vi "Main.vi"() -> ()   [LabVIEW 2017]
uses:
  states.ctl
  data.ctl
panel:
  in  "Save Config":bool caption="Save"
  in  "Log While\nCharging":enum32{"No Selection", " Yes", " No"}(radio) caption="Radio Buttons"
  in  "Sample\nRate":T1(radio) caption="Radio Buttons"
  in  "Load Config":bool caption="Config"
  in  "Download All (Single)":bool
  in  "Download File Path":path
  in  "Download":bool
  in  "View File":bool
  in  "File Selection":u16(ring)
  in  "Drifter Selection":u16(ring) items=["Drifter Number: 000 (10.0.1.3)", "Drifter Number: 001 (10.0.1.6)"]
  out "Info Box":string
  in  "Save Table":bool
  in  "Load Table":bool
  in  "MAC & Name":string[][](table)=[["", ""], ["", ""]]
  in  "Find Drifters":bool
  in  "List Data Files":bool
  in  "Stop":bool
  # "GPS Drifter Interface Software"
  # "Wolfson School of Mechanical, Electrical and Manufacturing Engineering"
  # "Thomas Quinn B224307 MEng Advanced Project 2017/2018"
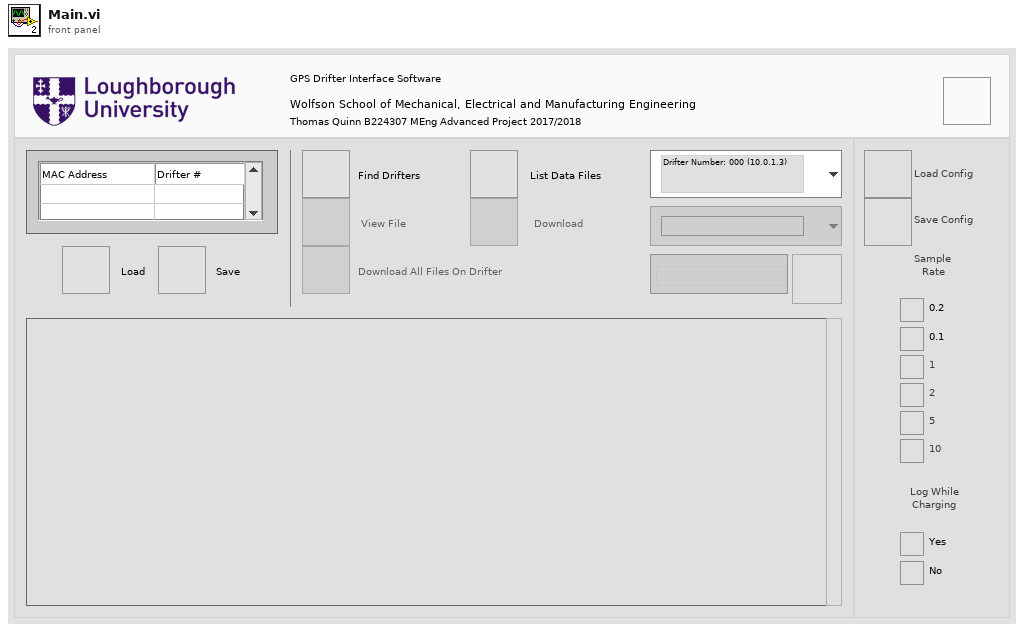
[diagram p1: front panel]
types:
  T1 = enum32{"No Selection", " 0.2", " 0.1", " 1", " 2", " 5", " 10"}
  T2 = enum8{"Enabled", "Disabled", "Disabled and Grayed Out"}
  T3 = typedef "data.ctl" = cluster{"Info Box":string, "MAC & Name Out":string[][], "Default Gateway":string, "Drfiter IP Addresses":string[][], "Network Map":string, "Drifter Selection":i32, "File Selection":i32, "Download File Path":path, "File Selection Strings":string[], "Sample Rate":enum32{"No Selection", " 0.2", " 0.1", " 1", " 2", " 5", " 10"}, "Log While Charging":enum32{"No Selection", " Yes", " No"}}
  T4 = typedef "states.ctl" = cluster{"Enum":enum16{"Stop", "Init", "List Data Files", "Find Default Gateway", "Save Table", "Load Table", "Ping Entire Network", "Network Map", "Match MAC Addresses", "Check IP Addresses", "Display IP Addresses", "File Selection", "View File", "Download File", "Download All (Single)", "Download File Path", "Load Config", "Save Config", "Update Config"}, "Message Data":variant}
  T5 = enum16{"Stop", "Init", "List Data Files", "Find Default Gateway", "Save Table", "Load Table", "Ping Entire Network", "Network Map", "Match MAC Addresses", "Check IP Addresses", "Display IP Addresses", "File Selection", "View File", "Download File", "Download All (Single)", "Download File Path", "Load Config", "Save Config", "Update Config"}
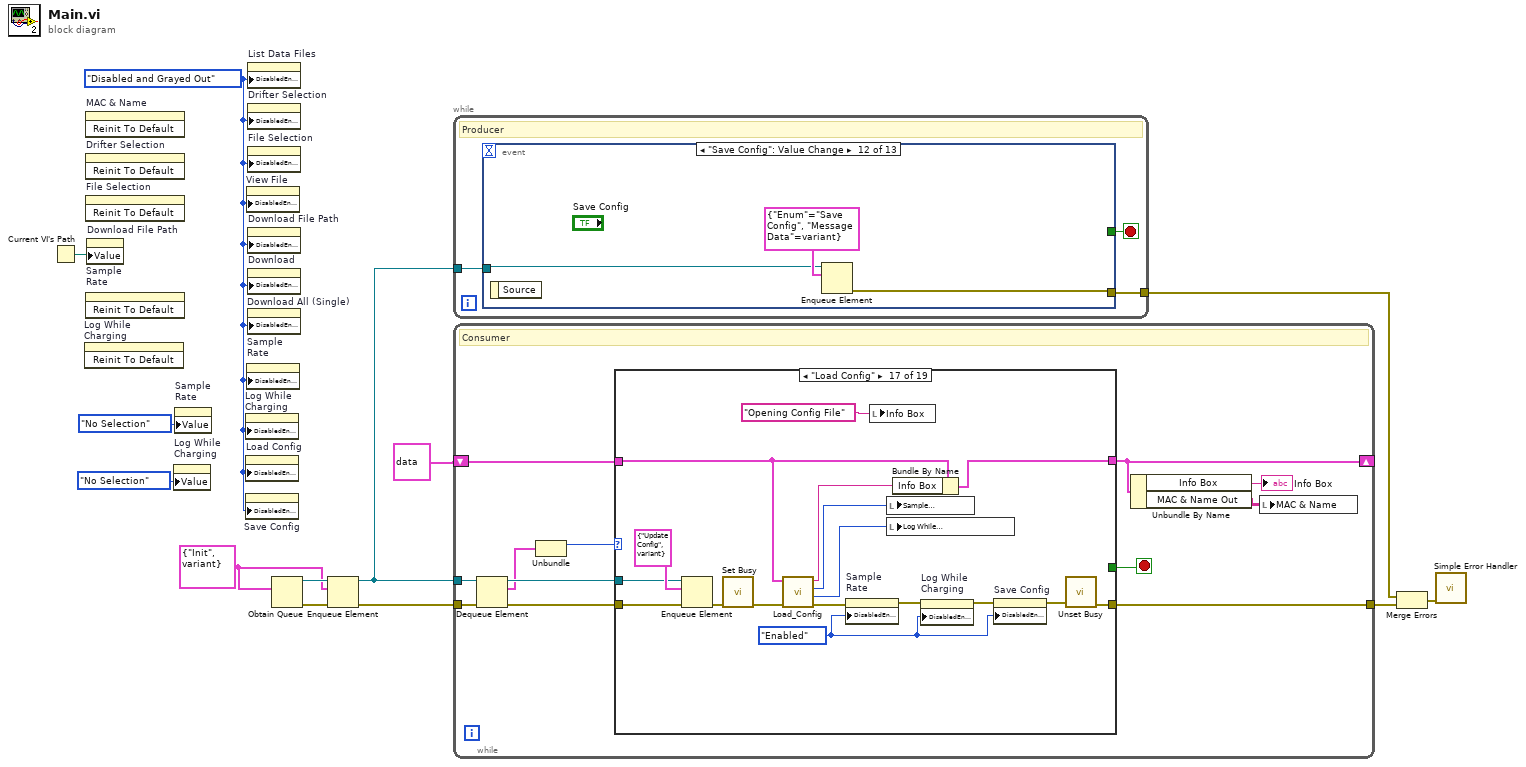
[diagram p0: block diagram]
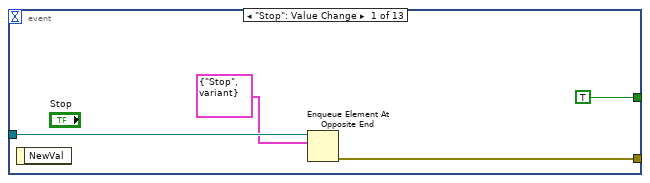
[diagram p2: hidden frame]
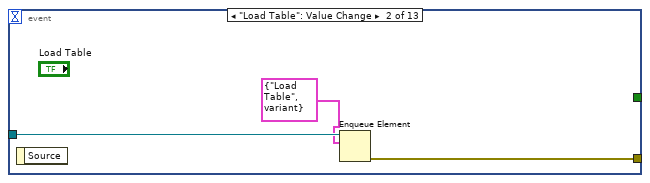
[diagram p3: hidden frame]
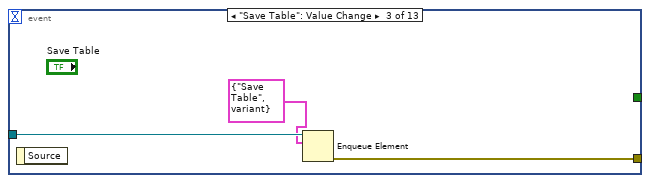
[diagram p4: hidden frame]
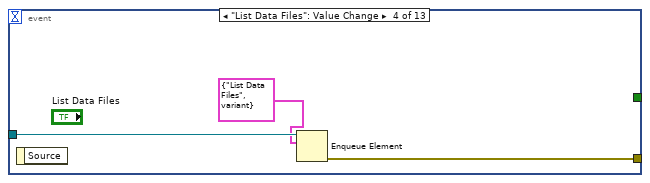
[diagram p5: hidden frame]
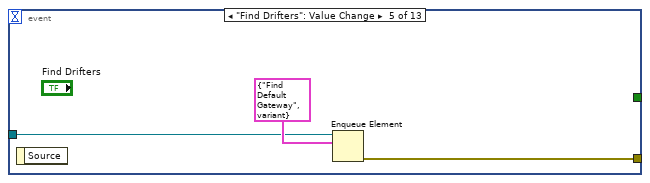
[diagram p6: hidden frame]
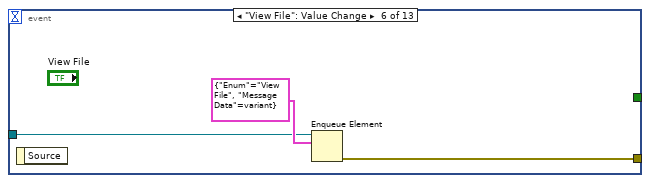
[diagram p7: hidden frame]
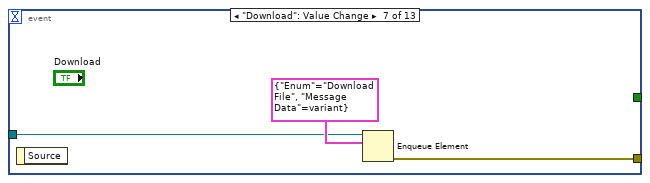
[diagram p8: hidden frame]
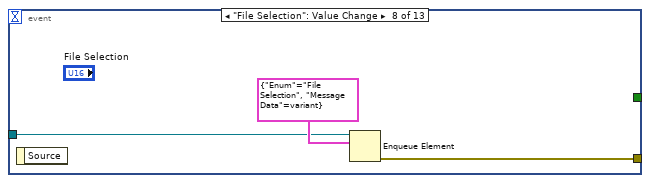
[diagram p9: hidden frame]
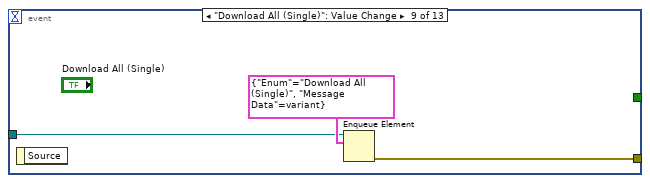
[diagram p10: hidden frame]
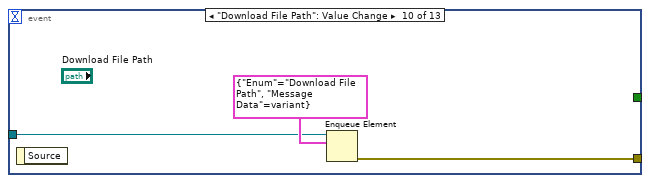
[diagram p11: hidden frame]
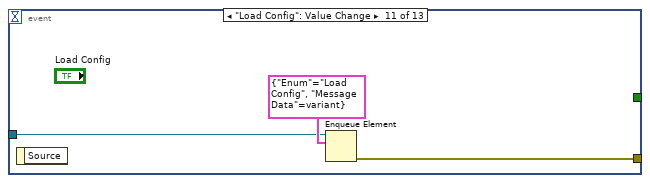
[diagram p12: hidden frame]
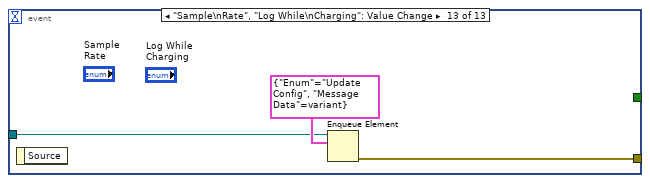
[diagram p13: hidden frame]
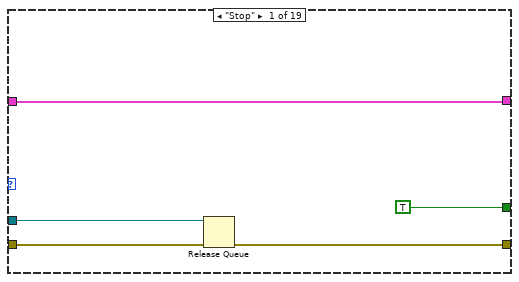
[diagram p14: hidden frame]
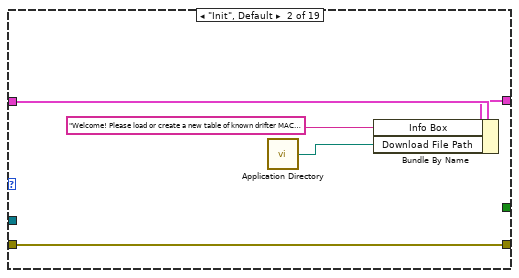
[diagram p15: hidden frame]
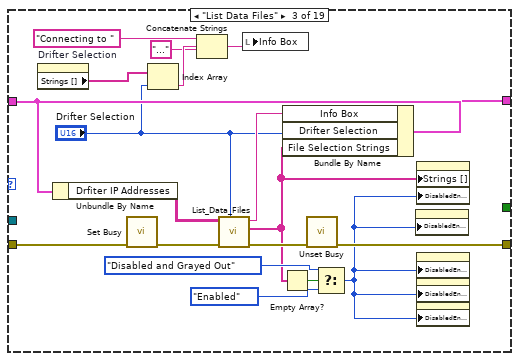
[diagram p16: hidden frame]
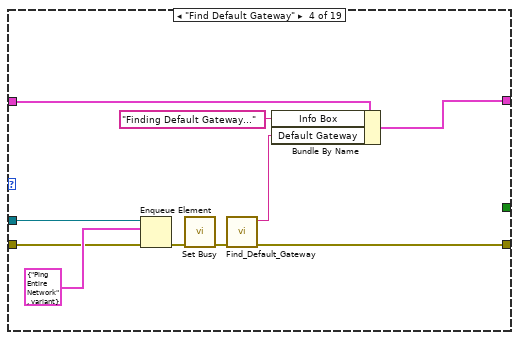
[diagram p17: hidden frame]
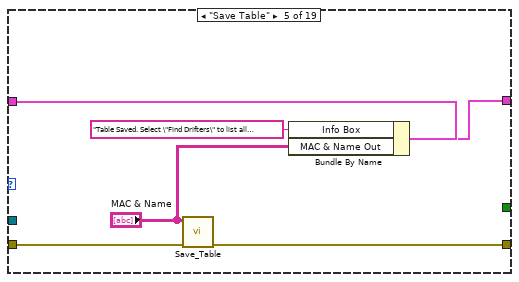
[diagram p18: hidden frame]
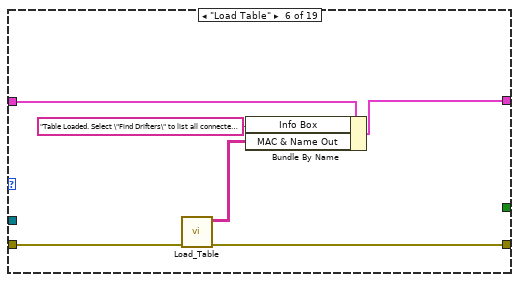
[diagram p19: hidden frame]
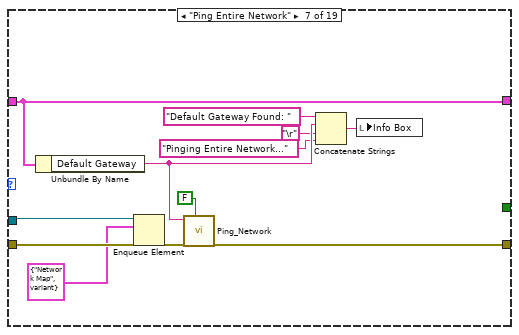
[diagram p20: hidden frame]
diagram:
  w1 = T2."Disabled and Grayed Out" ("Disabled")
  w6 = T4 {"Enum"=enum."Init", "Message Data"=variant}
  n1 = Current VI's Path() -> (path=w4:path)
  n2 = invoke on="Log While\nCharging" class="RadioBtnsControl (strict)" method="Reinit To Default"() -> ()  [unwired: 3 in, 3 out]
  n3 = invoke on="MAC & Name" class="Tbl (strict)" method="Reinit To Default"() -> ()  [unwired: 3 in, 3 out]
  n4 = invoke on="Drifter Selection" class="Ring (strict)" method="Reinit To Default"() -> ()  [unwired: 3 in, 3 out]
  n5 = invoke on="File Selection" class="Ring (strict)" method="Reinit To Default"() -> ()  [unwired: 3 in, 3 out]
  n6 = invoke on="Sample\nRate" class="RadioBtnsControl (strict)" method="Reinit To Default"() -> ()  [unwired: 3 in, 3 out]
  n7 = property on="Download File Path" class="Path"("Value"=w4) -> ()  [unwired: 2 in, 2 out]
  n8 = property on="Log While\nCharging" class="RadioBtnsControl (strict)"("Value"=enum32{"No Selection", " Yes", " No"}."No Selection" ("Log While\nCharging")) -> ()  [unwired: 2 in, 2 out]
  n9 = property on="Sample\nRate" class="RadioBtnsControl (strict)"("Value"=T1."No Selection" ("Sample\nRate")) -> ()  [unwired: 2 in, 2 out]
  n10 = property on="Log While\nCharging" class="RadioBtnsControl (strict)"("DisabledEnum"=w1) -> ()  [unwired: 2 in, 2 out]
  n11 = property on="Load Config" class="Bool"("DisabledEnum"=w1) -> ()  [unwired: 2 in, 2 out]
  n12 = property on="Save Config" class="Bool"("DisabledEnum"=w1) -> ()  [unwired: 2 in, 2 out]
  n13 = property on="View File" class="Bool"("DisabledEnum"=w1) -> ()  [unwired: 2 in, 2 out]
  n14 = property on="Sample\nRate" class="RadioBtnsControl (strict)"("DisabledEnum"=w1) -> ()  [unwired: 2 in, 2 out]
  n15 = property on="List Data Files" class="Bool"("DisabledEnum"=w1) -> ()  [unwired: 2 in, 2 out]
  n16 = property on="Drifter Selection" class="Ring (strict)"("DisabledEnum"=w1) -> ()  [unwired: 2 in, 2 out]
  n17 = property on="File Selection" class="Ring (strict)"("DisabledEnum"=w1) -> ()  [unwired: 2 in, 2 out]
  n18 = property on="Download File Path" class="Path"("DisabledEnum"=w1) -> ()  [unwired: 2 in, 2 out]
  n19 = property on="Download" class="Bool"("DisabledEnum"=w1) -> ()  [unwired: 2 in, 2 out]
  n20 = property on="Download All (Single)" class="Bool"("DisabledEnum"=w1) -> ()  [unwired: 2 in, 2 out]
  n21 = Obtain Queue(element data type=w6) -> (queue out=w10:refnum<queue>, error out=w11:errorcluster)  [unwired: 4 in, 1 out]
  n22 = Enqueue Element(queue=w10, element=w6, error in (no error)=w11) -> (queue out=w8:refnum<queue>, error out=w9:errorcluster)  [unwired: 1 in, 1 out]
  n23 = while {
    tunnel: w8 -> [w16]
    tunnel: [w14] -> w12
    stop <- w15 stop-if-true
    # "Producer"
    n24 = event shown="[11] \"Save Config\": Value Change" {
      selector: _ -> [_ _ _ _ _ _ _ _ _ _ _ _ _]
      dyn-events: _ -> [_ _ _ _ _ _ _ _ _ _ _ _ _]
      timeout: _ -> [_ _ _ _ _ _ _ _ _ _ _ _ _]
      tunnel: [TRUE _ _ _ _ _ _ _ _ _ _ _ _] -> w15
      tunnel: w16 -> [w20 w22 w25 w28 w31 w33 w36 w39 w42 w45 w48 w51 w54]
      tunnel: [w19 w23 w26 w29 w30 w34 w37 w40 w43 w46 w49 w52 w55] -> w14
      event "Stop": Value Change {
        n25 = event-data() -> ()  [unwired: 1 in, 1 out]
        n26 = Enqueue Element At Opposite End(queue=w20, element=T4 {"Enum"=enum."Stop", "Message Data"=variant}) -> (error out=w19:errorcluster)  [unwired: 2 in, 2 out]
      }
      event "Load Table": Value Change {
        n27 = event-data() -> ()  [unwired: 1 in, 1 out]
        n28 = Enqueue Element(queue=w22, element=T4 {"Enum"=enum."Load Table", "Message Data"=variant}) -> (error out=w23:errorcluster)  [unwired: 2 in, 2 out]
      }
      event "Save Table": Value Change {
        n29 = event-data() -> ()  [unwired: 1 in, 1 out]
        n30 = Enqueue Element(queue=w25, element=T4 {"Enum"=enum."Save Table", "Message Data"=variant}) -> (error out=w26:errorcluster)  [unwired: 2 in, 2 out]
      }
      event "List Data Files": Value Change {
        n31 = event-data() -> ()  [unwired: 1 in, 1 out]
        n32 = Enqueue Element(queue=w28, element=T4 {"Enum"=enum."List Data Files", "Message Data"=variant}) -> (error out=w29:errorcluster)  [unwired: 2 in, 2 out]
      }
      event "Find Drifters": Value Change {
        n33 = event-data() -> ()  [unwired: 1 in, 1 out]
        n34 = Enqueue Element(queue=w31, element=T4 {"Enum"=enum."Find Default Gateway", "Message Data"=variant}) -> (error out=w30:errorcluster)  [unwired: 2 in, 2 out]
      }
      event "View File": Value Change {
        n35 = event-data() -> ()  [unwired: 1 in, 1 out]
        n36 = Enqueue Element(queue=w33, element=T4 {"Enum"=enum."View File", "Message Data"=variant}) -> (error out=w34:errorcluster)  [unwired: 2 in, 2 out]
      }
      event "Download": Value Change {
        n37 = event-data() -> ()  [unwired: 1 in, 1 out]
        n38 = Enqueue Element(queue=w36, element=T4 {"Enum"=enum."Download File", "Message Data"=variant}) -> (error out=w37:errorcluster)  [unwired: 2 in, 2 out]
      }
      event "File Selection": Value Change {
        n39 = event-data() -> ()  [unwired: 1 in, 1 out]
        n40 = Enqueue Element(queue=w39, element=T4 {"Enum"=enum."File Selection", "Message Data"=variant}) -> (error out=w40:errorcluster)  [unwired: 2 in, 2 out]
      }
      event "Download All (Single)": Value Change {
        n41 = event-data() -> ()  [unwired: 1 in, 1 out]
        n42 = Enqueue Element(queue=w42, element=T4 {"Enum"=enum."Download All (Single)", "Message Data"=variant}) -> (error out=w43:errorcluster)  [unwired: 2 in, 2 out]
      }
      event "Download File Path": Value Change {
        n43 = event-data() -> ()  [unwired: 1 in, 1 out]
        n44 = Enqueue Element(queue=w45, element=T4 {"Enum"=enum."Download File Path", "Message Data"=variant}) -> (error out=w46:errorcluster)  [unwired: 2 in, 2 out]
      }
      event "Load Config": Value Change {
        n45 = event-data() -> ()  [unwired: 1 in, 1 out]
        n46 = Enqueue Element(queue=w48, element=T4 {"Enum"=enum."Load Config", "Message Data"=variant}) -> (error out=w49:errorcluster)  [unwired: 2 in, 2 out]
      }
      event "Save Config": Value Change {
        n47 = event-data() -> ()  [unwired: 1 in, 1 out]
        n48 = Enqueue Element(queue=w51, element=T4 {"Enum"=enum."Save Config", "Message Data"=variant}) -> (error out=w52:errorcluster)  [unwired: 2 in, 2 out]
      }
      event "Sample\nRate", "Log While\nCharging": Value Change {
        n49 = event-data() -> ()  [unwired: 1 in, 1 out]
        n50 = Enqueue Element(queue=w54, element=T4 {"Enum"=enum."Update Config", "Message Data"=variant}) -> (error out=w55:errorcluster)  [unwired: 2 in, 2 out]
      }
    }
  }
  n51 = while {
    tunnel: w8 -> [w66]
    tunnel: w9 -> [w67]
    tunnel: [w68] -> w13
    shift-right: [w59] -> _
    shift-left: T3 {"Info Box"="", "MAC & Name Out"=[], "Default Gateway"="", "Drfiter IP Addresses"=[], "Network Map"="", "Drifter Selection"=0, "File Selection"=0, "Download File Path"=path "", "File Selection Strings"=[], "Sample Rate"=enum." 0.2", "Log While Charging"=enum." Yes"} ("Data") -> [w60]
    stop <- w61 stop-if-true
    # "Consumer"
    n52 = Dequeue Element(queue=w66, error in (no error)=w67) -> (queue out=w65:refnum<queue>, element=w63:T4, error out=w64:errorcluster)  [unwired: 1 in, 1 out]
    n53 = Unbundle(w63) -> ("Enum"=w62:T5)  [unwired: 1 out]
    n54 = case "Message Cases" shown="\"Load Config\"" w62 {
      tunnel: w65 -> [w71 _ _ w105 _ _ w126 w137 w147 w164 _ _ _ _ _ _ w220 w237 _]
      tunnel: w64 -> [w73 w78 w84 w106 w113 w119 w128 w139 w148 w163 w172 w183 w193 w201 w209 w219 w222 w238 w254]
      tunnel: [w72 w78 w81 w98 w112 w118 w129 w141 w151 w160 w168 w180 w191 w201 w210 w219 w232 w244 w254] -> w68
      tunnel: [TRUE _ _ _ _ _ _ _ _ _ _ _ _ _ _ _ _ _ _] -> w61
      tunnel: w60 -> [w69 w77 w91 w101 w111 w117 w125 w136 w144 w158 w169 w175 w189 w199 w208 w217 w231 w247 w253]
      tunnel: [w69 w76 w90 w102 w110 w116 w125 w135 w143 w157 w173 w185 w189 w198 w208 w218 w230 w246 w252] -> w59
      frame "Stop" {
        n55 = Release Queue(queue=w71, error in (no error)=w73) -> (error out=w72:errorcluster)  [unwired: 1 in, 2 out]
      }
      frame "Init", Default {
        n56 = call <vilib>:"Application Directory.vi"() -> ("Application Directory"=w74:path)
        n57 = Bundle By Name(cluster=w77, "Info Box"="Welcome! Please load or create a new table of known drifter MAC addresses and associated number.", "Download File Path"=w74) -> (w76:T3)
      }
      frame "List Data Files" {
        n58 = property on="Drifter Selection" class="Ring (strict)"() -> ("Strings []"=w94:string[])  [unwired: 2 in, 2 out]
        n59 = Unbundle By Name(w91) -> ("Drfiter IP Addresses"=w97:string[][])
        n60 = call <vilib>:"Set Busy.vi"("error in (no error)"=w84) -> ("error out"=w83:errorcluster)  [unwired: 9 in, 1 out]
        n61 = Index Array(array=w94, index="Drifter Selection") -> (element=w93:string)
        n62 = Concatenate Strings("Connecting to " ("Info Box"), w93, "..." ("string")) -> (w96:string)
        n63 = call "List_Data_Files.vi"("Drifter"="Drifter Selection", "Error In"=w83, "Drfiter IP Addresses"=w97) -> ("Error Out"=w82:errorcluster, "File List Array"=w80:string[], "File List"=w89:string)  [unwired: 6 in]
        n64 = local write "Info Box"(w96) -> ()
        n65 = Empty Array?(array=w80) -> (empty?=w88:bool)
        n66 = Bundle By Name(cluster=w91, "Info Box"=w89, "Drifter Selection"="Drifter Selection", "File Selection Strings"=w80) -> (w90:T3)
        n67 = call <vilib>:"Unset Busy.vi"("error in (no error)"=w82) -> ("error out"=w81:errorcluster)  [unwired: 10 in]
        n68 = Select(t=T2."Disabled and Grayed Out" ("Disabled"), s=w88, f=T2."Enabled" ("Disabled")) -> (s? t:f=w79:T2)
        n69 = property on="Download File Path" class="Path"("DisabledEnum"=w79) -> ()  [unwired: 2 in, 2 out]
        n70 = property on="File Selection" class="Ring (strict)"("Strings []"=w80, "DisabledEnum"=w79) -> ()  [unwired: 2 in, 2 out]
        n71 = property on="View File" class="Bool"("DisabledEnum"=w79) -> ()  [unwired: 2 in, 2 out]
        n72 = property on="Download" class="Bool"("DisabledEnum"=w79) -> ()  [unwired: 2 in, 2 out]
        n73 = property on="Download All (Single)" class="Bool"("DisabledEnum"=w79) -> ()  [unwired: 2 in, 2 out]
      }
      frame "Find Default Gateway" {
        n74 = Enqueue Element(queue=w105, element=T4 {"Enum"=enum."Ping Entire Network", "Message Data"=variant}, error in (no error)=w106) -> (error out=w104:errorcluster)  [unwired: 1 in, 2 out]
        n75 = call <vilib>:"Set Busy.vi"("error in (no error)"=w104) -> ("error out"=w103:errorcluster)  [unwired: 9 in, 1 out]
        n76 = call "Find_Default_Gateway.vi"("Error In"=w103) -> ("Error Out"=w98:errorcluster, "Default Gateway"=w99:string)  [unwired: 9 in]
        n77 = Bundle By Name(cluster=w101, "Info Box"="Finding Default Gateway..." ("Terminal Output"), "Default Gateway"=w99) -> (w102:T3)
      }
      frame "Save Table" {
        n78 = call "Save_Table.vi"("Error In"=w113, "MAC & Name In"="MAC & Name") -> ("Error Out"=w112:errorcluster)  [unwired: 9 in]
        n79 = Bundle By Name(cluster=w111, "Info Box"="Table Saved. Select \"Find Drifters\" to list all connected drifters.", "MAC & Name Out"="MAC & Name") -> (w110:T3)
      }
      frame "Load Table" {
        n80 = call "Load_Table.vi"("Error In"=w119) -> ("Error Out"=w118:errorcluster, "MAC & Name Out"=w115:string[][])  [unwired: 9 in]
        n81 = Bundle By Name(cluster=w117, "Info Box"="Table Loaded. Select \"Find Drifters\" to list all connected drifters.", "MAC & Name Out"=w115) -> (w116:T3)
      }
      frame "Ping Entire Network" {
        n82 = Unbundle By Name(w125) -> ("Default Gateway"=w122:string)
        n83 = Enqueue Element(queue=w126, element=T4 {"Enum"=enum."Network Map", "Message Data"=variant}) -> ()  [unwired: 2 in, 3 out]
        n84 = call "Ping_Network.vi"("IP/Default Gateway (T/F)"=FALSE, "Error In"=w128, "Default Gateway/IP"=w122) -> ("Error Out"=w129:errorcluster)  [unwired: 7 in, 1 out]
        n85 = Concatenate Strings("Default Gateway Found: " ("Info Box"), w122, "\r", "Pinging Entire Network..." ("Info Box")) -> (w124:string)
        n86 = local write "Info Box"(w124) -> ()
      }
      frame "Network Map" {
        n87 = Enqueue Element(queue=w137, element=T4 {"Enum"=enum."Match MAC Addresses", "Message Data"=variant}, error in (no error)=w139) -> (error out=w138:errorcluster)  [unwired: 1 in, 2 out]
        n88 = call "Network_Map_(WIN).vi"("Error In"=w138) -> ("Error Out"=w141:errorcluster, "Terminal Output"=w132:string)  [unwired: 9 in]
        n89 = Concatenate Strings("Network Map Generated. Matching MAC addresses and validating IP addresses..." ("string"), "\r\n", w132) -> (w134:string)
        n90 = Bundle By Name(cluster=w136, "Info Box"=w134, "Network Map"=w132) -> (w135:T3)
      }
      frame "Match MAC Addresses" {
        n91 = Unbundle By Name(w144) -> ("MAC & Name Out"=w145:string[][], "Network Map"=w146:string)
        n92 = Enqueue Element(queue=w147, element=T4 {"Enum"=enum."Check IP Addresses", "Message Data"=variant}, error in (no error)=w148) -> (error out=w149:errorcluster)  [unwired: 1 in, 2 out]
        n93 = call "Match_MAC.vi"("MAC & Name In"=w145, "Error In"=w149, "Network Map In"=w146) -> ("Error Out"=w151:errorcluster, "Drfiter IP Addresses Out"=w142:string[][])  [unwired: 7 in]
        n94 = Bundle By Name(cluster=w144, "Drfiter IP Addresses"=w142) -> (w143:T3)
      }
      frame "Check IP Addresses" {
        n95 = Unbundle By Name(w158) -> ("Drfiter IP Addresses"=w159:string[][])
        n96 = Enqueue Element(queue=w164, element=T4 {"Enum"=enum."Display IP Addresses", "Message Data"=variant}, error in (no error)=w163) -> (error out=w162:errorcluster)  [unwired: 1 in, 2 out]
        n97 = call "Check_IP.vi"("Error In"=w162, "Drfiter IP Addresses In"=w159) -> ("Error Out"=w161:errorcluster, "Drfiter IP Addresses Out"=w154:string[][])  [unwired: 8 in]
        n98 = call <vilib>:"Unset Busy.vi"("error in (no error)"=w161) -> ("error out"=w160:errorcluster)  [unwired: 10 in]
        n99 = Bundle By Name(cluster=w158, "Drfiter IP Addresses"=w154) -> (w157:T3)
        n100 = Empty Array?(array=w154) -> (empty?=w155:bool)
        n101 = Select(t=T2."Disabled and Grayed Out", s=w155, f=T2."Enabled" ("Disabled")) -> (s? t:f=w152:T2)
        n102 = property on="List Data Files" class="Bool"("DisabledEnum"=w152) -> ()  [unwired: 2 in, 2 out]
        n103 = property on="Drifter Selection" class="Ring (strict)"("DisabledEnum"=w152) -> ()  [unwired: 2 in, 2 out]
      }
      frame "Display IP Addresses" {
        n104 = call "Display_IP_Addresses.vi"("Error In"=w172, "Data"=w169) -> ("Error Out"=w167:errorcluster, "Menu String"=w170:string[], "Output Text"=w171:string)  [unwired: 7 in]
        n105 = property on="Drifter Selection" class="Ring (strict)"("Strings []"=w170) -> ()  [unwired: 2 in, 2 out]
        n106 = Bundle By Name(cluster=w169, "Info Box"=w171) -> (w173:T3)
        n107 = property on="Load Config" class="Bool"(error in=w167, "DisabledEnum"=T2."Enabled" ("Disabled")) -> (error out=w168:errorcluster)  [unwired: 1 in, 1 out]
      }
      frame "View File" {
        n108 = call <vilib>:"Set Busy.vi"("error in (no error)"=w183) -> ("error out"=w182:errorcluster)  [unwired: 9 in, 1 out]
        n109 = Unbundle By Name(w175) -> ("File Selection"=w174:i32)
        n110 = property on="File Selection" class="Ring (strict)"() -> ("Strings []"=w176:string[])  [unwired: 2 in, 2 out]
        n111 = call "View_File.vi"("File Selection"=w174, "Error In"=w182, "Data"=w175) -> ("Error Out"=w181:errorcluster, "File Contents"=w184:string)  [unwired: 7 in]
        n112 = Index Array(array=w176, index=w174) -> (element=w178:string)
        n113 = Concatenate Strings("Opening " ("Info Box"), w178) -> (w179:string)
        n114 = call <vilib>:"Unset Busy.vi"("error in (no error)"=w181) -> ("error out"=w180:errorcluster)  [unwired: 10 in]
        n115 = Bundle By Name(cluster=w175, "Info Box"=w184) -> (w185:T3)
        n116 = local write "Info Box"(w179) -> ()
      }
      frame "Download File" {
        n117 = Unbundle By Name(w189) -> ("File Selection"=w186:i32, "Download File Path"=w188:path)
        n118 = property on="File Selection" class="Ring (strict)"() -> ("Strings []"=w195:string[])  [unwired: 2 in, 2 out]
        n119 = call <vilib>:"Set Busy.vi"("error in (no error)"=w193) -> ("error out"=w192:errorcluster)  [unwired: 9 in, 1 out]
        n120 = Index Array(array=w195, index=w186) -> (element=w196:string)
        n121 = call "Download_All_(Single).vi"("File Selection"=w186, "error in (no error)"=w192, "Data"=w189, "File Path Control"=w188) -> ("error out"=w190:errorcluster)  [unwired: 7 in]
        n122 = Concatenate Strings("Downloading " ("Info Box"), w196, "from current drifter." ("string")) -> (w197:string)
        n123 = local write "Info Box"(w197) -> ()
        n124 = call <vilib>:"Unset Busy.vi"("error in (no error)"=w190) -> ("error out"=w191:errorcluster)  [unwired: 10 in]
      }
      frame "File Selection" {
        n125 = local read "File Selection"() -> (w200:u16)
        n126 = Bundle By Name(cluster=w199, "File Selection"=w200) -> (w198:T3)
      }
      frame "Download All (Single)" {
        n127 = call <vilib>:"Set Busy.vi"("error in (no error)"=w209) -> ("error out"=w206:errorcluster)  [unwired: 9 in, 1 out]
        n128 = Unbundle By Name(w208) -> ("Download File Path"=w207:path)
        n129 = property on="File Selection" class="Ring (strict)"(error in=w206) -> (error out=w205:errorcluster, "NumItems"=w203:u32)  [unwired: 1 in, 1 out]
        n130 = for {
          N: w203 -> [_]
          tunnel: w208 -> [w215]
          tunnel: w207 -> [w214]
          shift-right: [w212] -> w204
          shift-left: w205 -> [w213]
          i -> [w211]
          n131 = call "Download_All_(Single).vi"("File Selection"=w211, "error in (no error)"=w213, "Data"=w215, "File Path Control"=w214) -> ("error out"=w212:errorcluster)  [unwired: 7 in]
        }
        n132 = local write "Info Box"("Downloading all data from current drifter.  " ("Info Box")) -> ()
        n133 = call <vilib>:"Unset Busy.vi"("error in (no error)"=w204) -> ("error out"=w210:errorcluster)  [unwired: 10 in]
      }
      frame "Download File Path" {
        n134 = local read "Download File Path"() -> (w216:path)
        n135 = Bundle By Name(cluster=w217, "Download File Path"=w216) -> (w218:T3)
      }
      frame "Load Config" {
        w224 = T2."Enabled" ("Disabled")
        n136 = Enqueue Element(queue=w220, element=T4 {"Enum"=enum."Update Config", "Message Data"=variant}, error in (no error)=w222) -> (error out=w221:errorcluster)  [unwired: 1 in, 2 out]
        n137 = call <vilib>:"Set Busy.vi"("error in (no error)"=w221) -> ("error out"=w233:errorcluster)  [unwired: 9 in, 1 out]
        n138 = call "Load_Config.vi"("Error In"=w233, "Data"=w231) -> ("Error Out"=w235:errorcluster, "Log While\nCharging"=w228:enum32{"No Selection", " Yes", " No"}, "Sample\nRate"=w227:T1, "File Contents"=w229:string)  [unwired: 6 in]
        n139 = property on="Sample\nRate" class="RadioBtnsControl (strict)"(error in=w235, "DisabledEnum"=w224) -> (error out=w236:errorcluster)  [unwired: 1 in, 1 out]
        n140 = local write "Info Box"("Opening Config File" ("Info Box")) -> ()
        n141 = local write "Sample\nRate"(w227) -> ()
        n142 = local write "Log While\nCharging"(w228) -> ()
        n143 = Bundle By Name(cluster=w231, "Info Box"=w229) -> (w230:T3)
        n144 = property on="Log While\nCharging" class="RadioBtnsControl (strict)"(error in=w236, "DisabledEnum"=w224) -> (error out=w226:errorcluster)  [unwired: 1 in, 1 out]
        n145 = property on="Save Config" class="Bool"(error in=w226, "DisabledEnum"=w224) -> (error out=w225:errorcluster)  [unwired: 1 in, 1 out]
        n146 = call <vilib>:"Unset Busy.vi"("error in (no error)"=w225) -> ("error out"=w232:errorcluster)  [unwired: 10 in]
      }
      frame "Save Config" {
        n147 = Enqueue Element(queue=w237, element=T4 {"Enum"=enum."Load Config", "Message Data"=variant}, error in (no error)=w238) -> (timed out?=w240:bool, error out=w239:errorcluster)  [unwired: 1 in, 1 out]
        n148 = call <vilib>:"Set Busy.vi"("error in (no error)"=w239, "disable click? (T)"=w240) -> ("error out"=w242:errorcluster)  [unwired: 8 in, 1 out]
        n149 = call "Create_Config.vi"("Error In"=w242, "Data"=w247) -> ("Error Out"=w248:errorcluster)  [unwired: 9 in]
        n150 = call "Save_Config.vi"("Error In"=w248, "Data"=w247) -> ("Error Out"=w243:errorcluster, "File Contents"=w245:string)  [unwired: 8 in]
        n151 = local write "Info Box"("Saving Config File" ("Info Box")) -> ()
        n152 = Bundle By Name(cluster=w247, "Info Box"=w245) -> (w246:T3)
        n153 = call <vilib>:"Unset Busy.vi"("error in (no error)"=w243) -> ("error out"=w244:errorcluster)  [unwired: 10 in]
      }
      frame "Update Config" {
        n154 = local read "Log While\nCharging"() -> (w250:enum32{"No Selection", " Yes", " No"})
        n155 = local read "Sample\nRate"() -> (w251:T1)
        n156 = Bundle By Name(cluster=w253, "Sample Rate"=w251, "Log While Charging"=w250) -> (w252:T3)
      }
    }
    n157 = Unbundle By Name(w59) -> ("Info Box"=→"Info Box":string, "MAC & Name Out"=w57:string[][])
    n158 = local write "MAC & Name"(w57) -> ()
  }
  n159 = Merge Errors(w12, w13) -> (w7:errorcluster)
  n160 = call <vilib>:"Simple Error Handler.vi"("error in (no error)"=w7) -> ()  [unwired: 4 in, 5 out]
